vi "8164B Set Power Units.vi"(8 "error in":errorcluster, 10 "Power Unit":T1, 11 "KeySight 8164B control in":T2) -> (0 "error out":errorcluster, 3 "KeySight 8164B control out":T2)   [LabVIEW 2018, in "KeySight 8164B LAN InstrLib.lvlib"]
uses:
  KeySight 8164B LAN InstrLib.lvlib
  typedefs/KeySight 8164B control.ctl
  typedefs/KeySight 8164B Power Unit.ctl
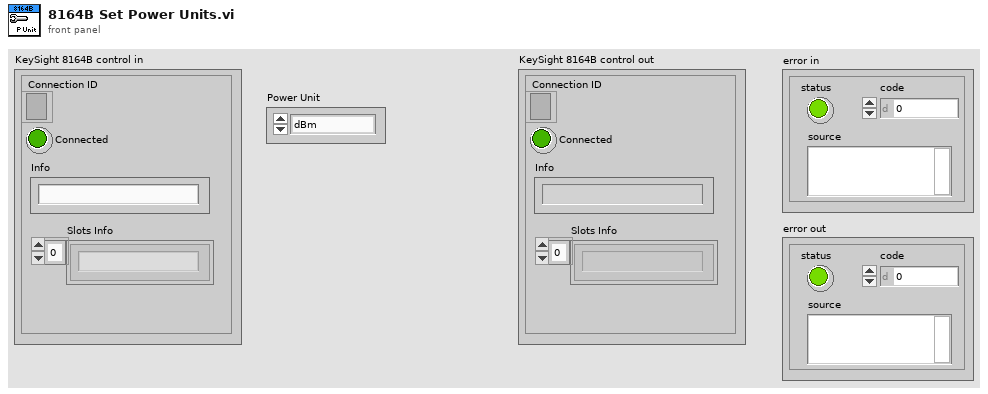
[diagram p1: front panel]
types:
  T1 = typedef "KeySight 8164B LAN InstrLib.lvlib/KeySight 8164B Power Unit.ctl" = enum16{"dBm", "Watt"}
  T2 = typedef "KeySight 8164B LAN InstrLib.lvlib/KeySight 8164B control.ctl" = cluster{"Connection ID":refnum<k5>, "Connected":bool, "Info":string, "Slots Info":string[]}
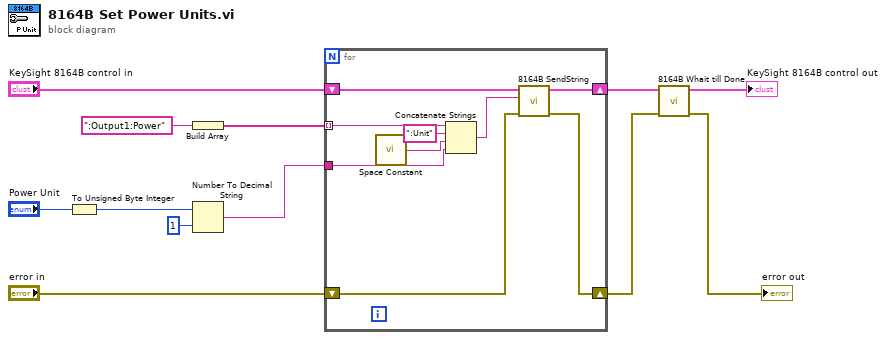
[diagram p0: block diagram]
diagram:
  n1 = To Unsigned Byte Integer(number="Power Unit") -> (unsigned 8bit integer=w7:u8)
  n2 = Build Array(":Output1:Power") -> (w9:string[])
  n3 = Number To Decimal String(number=w7, width (-)=i16 1) -> (decimal integer string=w5:string)
  n4 = for {
    shift-right: [w20] -> w4
    shift-left: "KeySight 8164B control in" -> [w21]
    shift-right: [w18] -> w2
    shift-left: "error in" -> [w19]
    tunnel: w5 -> [w14]
    tunnel: w9 -> [w17] mode=indexing
    n5 = call <vilib>:"Space Constant.vi"() -> ("String"=w15:string)
    n6 = Concatenate Strings(w17, ":Unit" ("string"), w15, w14) -> (w13:string)
    n7 = call "8164B SendString.vi"("error in"=w19, "CMD"=w13, "KeySight 8164B control in"=w21) -> ("error out"=w18:errorcluster, "KeySight 8164B control out"=w20:T2)  [unwired: 7 in]
  }
  n8 = call "8164B Whait till Done.vi"("error in"=w2, "KeySight 8164B control in"=w4) -> ("error out"=→"error out":errorcluster, "KeySight 8164B control out"=→"KeySight 8164B control out":T2)  [unwired: 8 in]
